vi "format set diag border.vi"(8 "error in (no error)":errorcluster, 10 "value":T1 items=["LXW_BORDER_NONE", "LXW_BORDER_THIN", "LXW_BORDER_MEDIUM", "LXW_BORDER_DASHED", "LXW_BORDER_DOTTED", "LXW_BORDER_THICK", "LXW_BORDER_DOUBLE", "LXW_BORDER_HAIR"], 11 "format":u32) -> (0 "error out":errorcluster)   [LabVIEW 2015, in "xlsxwriter.lvlib"]
doc: "void format_set_diag_border(lxw_format format, uint8_t value);"
uses:
  xlsxwriter.lvlib
  Controls/lxw_border_style.ctl
  xlsxwriter.dll
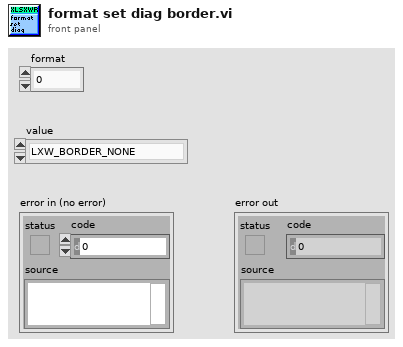
[diagram p1: front panel]
types:
  T1 = typedef "lxw_border_style.ctl" = u8
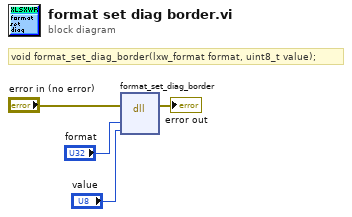
[diagram p0: block diagram]
diagram:
  # "void format_set_diag_border(lxw_format format, uint8_t value);"
  n1 = dll-call lib="C:/Users/WDAGUtilityAccount/Desktop/Labview_Example-win32/xlsxwriter.*" fn="format_set_diag_border"(error in="error in (no error)", "format"="format", "value"="value") -> (error out=→"error out":errorcluster)  [unwired: 5 in, 1 out]
